vi "Disconnect.vi"(0 "SLSC Local in":refnum<class "SLSC Local.lvclass">, 5 "devices":refnum<k21>="$DefaultDevices", 11 "error in (no error)":errorcluster) -> (4 "SLSC Local out":refnum<class "SLSC Local.lvclass">, 15 "error out":errorcluster)   [LabVIEW 2015, in "SLSC Local.lvclass"]
uses:
  SLSC Local.lvclass
  <vilib>/SLSC/SLSC.lvlib
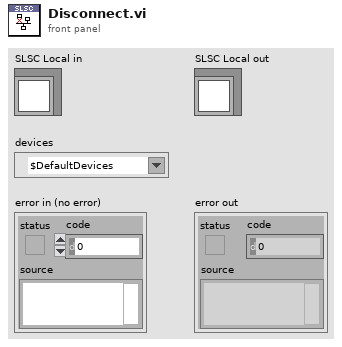
[diagram p1: front panel]
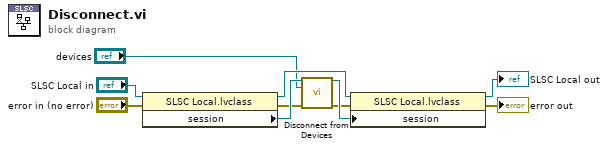
[diagram p0: block diagram]
diagram:
  n1 = property class="SLSC Local.lvclass"(reference="SLSC Local in", error in="error in (no error)") -> (reference out=w9:refnum<class "SLSC Local.lvclass">, error out=w6:errorcluster, "session"=w7:refnum<k21>)
  n2 = call <vilib>:"Disconnect from Devices.vi"("session in"=w7, "devices"="devices", "error in (no error)"=w6) -> ("session out"=w5:refnum<k21>, "error out"=w4:errorcluster)  [unwired: 11 in]
  n3 = property class="SLSC Local.lvclass"(reference=w9, error in=w4, "session"=w5) -> (reference out=→"SLSC Local out":refnum<class "SLSC Local.lvclass">, error out=→"error out":errorcluster)
